vi "galvo_ETL_offset_config.vi"(6 "sampling info":cluster{"Fs":dbl, "#s":dbl}={"Fs"=1000.0, "#s"=1000.0} {"Fs" format="%.2p"}, 8 "error in (no error)":errorcluster, 9 "ETL offset":dbl=2.0, 10 "Galvo offset":dbl, 11 "task/channels in":refnum<k21>) -> (0 "error out":errorcluster, 3 "task out":refnum<k21>)   [LabVIEW 2017]
uses:
  <vilib>/DAQmx/write.llb/DAQmx Write (Analog 1D Wfm NChan NSamp).vi
  <vilib>/DAQmx/miscellaneous.llb/DAQmx Fill In Error Info.vi
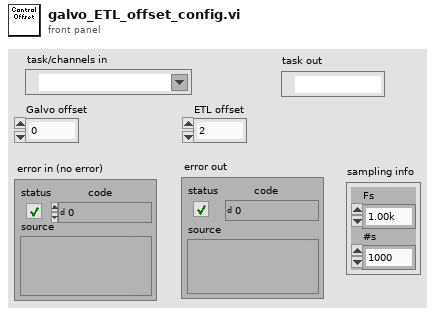
[diagram p1: front panel]
types:
  T1 = cluster{"frequency":dbl, "amplitude":dbl, "offset":dbl, "phase":dbl}
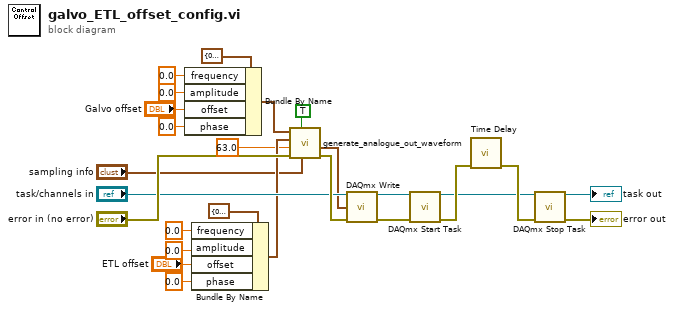
[diagram p0: block diagram]
diagram:
  n1 = Bundle By Name(cluster=T1 {"frequency"=0.0, "amplitude"=0.0, "offset"=0.0, "phase"=0.0}, "frequency"=0.0, "amplitude"=0.0, "offset"="Galvo offset", "phase"=0.0) -> (w8:T1)
  n2 = Bundle By Name(cluster=T1 {"frequency"=0.0, "amplitude"=0.0, "offset"=0.0, "phase"=0.0}, "frequency"=0.0, "amplitude"=0.0, "offset"="ETL offset", "phase"=0.0) -> (w6:T1)
  n3 = call "generate_analogue_out_waveform.vi"("sampling info"="sampling info", "Reset signal"=TRUE, "error in (no error)"="error in (no error)", "Camera start trigger phase"=63.0, "Vetl sine"=w6, "Vgalvo sine"=w8) -> ("error out"=w24:errorcluster, "Waveform Graph"=w10:waveform(dbl)[])  [unwired: 4 in]
  n4 = call-poly <vilib>:"DAQmx Write.vi"("task/channels in"="task/channels in", "data"=w10, "error in"=w24) -> ("task out"=w26:refnum<k21>, "error out"=w25:errorcluster)  [unwired: 10 in, 1 out]
  n5 = call <vilib>:"DAQmx Start Task.vi"("task/channels in"=w26, "error in"=w25) -> ("task out"=w2:refnum<k21>, "error out"=w14:errorcluster)  [unwired: 12 in]
  n6 = call "Time Delay"("error in (no error)"=w14) -> ("error out"=w13:errorcluster)  [unwired: 10 in]
  n7 = call <vilib>:"DAQmx Stop Task.vi"("task/channels in"=w2, "error in"=w13) -> ("task out"=→"task out":refnum<k21>, "error out"=→"error out":errorcluster)  [unwired: 12 in]
